vi "Read PWM-Delay-URLs.vi"(8 "error in (no error)":errorcluster, 11 "BNT_DAQmx-MCSV-DOPWM in":refnum<class "BNT_DAQmx-MCSV-DOPWM.lvclass">) -> (0 "error out":errorcluster, 2 "PWM-Delay-URLs":string[](array[string]), 3 "BNT_DAQmx-MCSV-DOPWM out":refnum<class "BNT_DAQmx-MCSV-DOPWM.lvclass">)   [LabVIEW 2019, in "BNT_DAQmx.lvlib" / "BNT_DAQmx-MCSV-DOPWM.lvclass"]
uses:
  BNT_DAQmx-MCSV-DOPWM.lvclass
  BNT_DAQmx-MCSV-DOPWM.lvclass/BNT_DAQmx-MCSV-DOPWM.ctl
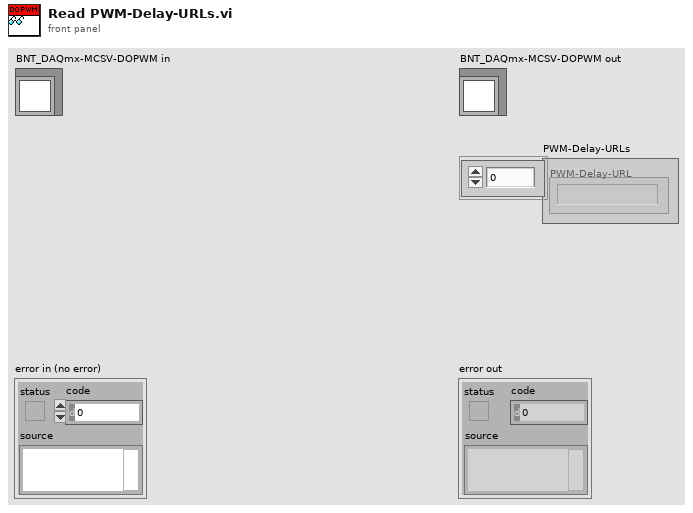
[diagram p1: front panel]
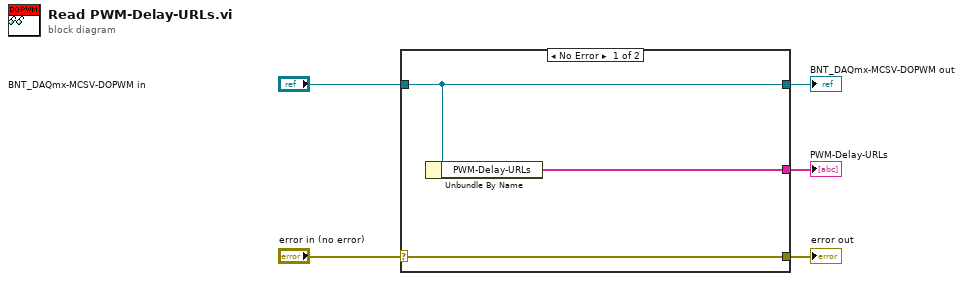
[diagram p0: block diagram]
diagram:
  n1 = case shown="No Error" "error in (no error)" {
    selector: "error in (no error)" -> [w8 w9]
    tunnel: [w8 w9] -> w4
    tunnel: [w7 w10] -> w2
    tunnel: "BNT_DAQmx-MCSV-DOPWM in" -> [w7 w10]
    tunnel: [w6 _] -> w1
    frame No Error {
      n2 = Unbundle By Name(w7) -> ("PWM-Delay-URLs"=w6:string[])
    }
    frame Error {
    }
  }
  "error out" <- w4
  "BNT_DAQmx-MCSV-DOPWM out" <- w2
  "PWM-Delay-URLs" <- w1
